vi "Keithley2450_and_24xx_plus_lockin_7_12_24.vi"() -> ()   [LabVIEW 2024]
uses:
  <vilib>/Analysis/1siggen.llb/Ramp Pattern by Delta.vi
  <vilib>/Utility/file.llb/Write Delimited Spreadsheet (string).vi
  <vilib>/Utility/file.llb/Write Delimited Spreadsheet (DBL).vi
  C:/Users/Public/OneDrive/Desktop/Keithley_2450_2470_1_4_0_LV2015_NewReadme2_2450-LV2015-1.4.0/Keithley 2450/Keithley 2450.lvlib
  <vilib>/Analysis/NI_AALBase.lvlib
  archive/Keithley 24XX/Keithley 24XX.lvlib
panel:
  out "XY Graph 2":cluster{dbl[], dbl[]}(graph)
  out "XY Graph":cluster{dbl[], dbl[]}(graph)
  in  "using 2400?":bool
  out "voltage 2410":dbl format="%0.2f"
  out "Current set voltage 2410":dbl
  in  "V stepsize 2410":dbl
  in  "start V 2410":dbl
  in  "End V 2410":dbl
  out "standard deviation current measured 2450":dbl=1.0551691053593696e-12 format="%0.5e"
  out "mean current measured 2450":dbl=3.19386155e-12 format="%0.5e"
  out "standard deviation current measured 2410":dbl format="%0.5e"
  out "mean current measured 2410":dbl format="%0.5e"
  in  "Compliance  Level 2410":dbl=1e-06
  in  "VISA resource name 2410":refnum<visa-resource-name>="GPIB0::24::INSTR"
  in  "Serial Configuration":T1={"Baud Rate"=9600, "Parity"=0, "Data Bits"=8, "Stop Bits"=10, "Flow Control"=0} {"Flow Control" items=["None", "XON/XOFF", "RTS/CTS", "XON/XOFF & RTS/CTS", "DTR/DSR", "XON/XOFF & DTR/DSR"]; "Stop Bits" items=["1.0"=10, "1.5"=15, "2.0"=20]; "Data Bits" items=["7"=7, "8"=8]; "Parity" items=["None", "Odd", "Even", "Mark", "Space"]; "Baud Rate" items=["300"=300, "600"=600, "1200"=1200, "2400"=2400, "4800"=4800, "9600"=9600, "19200"=19200]}
  in  "Wait for Current Meas":u32=100
  in  "Number of Current Meas":u32=20
  in  "Loop?":bool=TRUE
  out "Current set voltage 2450":dbl
  in  "V stepsize 2450":dbl=0.5
  in  "start V 2450":dbl
  in  "End V 2450":dbl=2.0
  in  "Wait for lock in meas (ms)":i32=2000
  in  "File Path":path=path "C:/Users/Public/OneDrive/Desktop/test.txt"
  out "错误输出":errorcluster={"status"=FALSE, "code"=1073676294, "source"="VISA Read in OE1022D_Query_Data.vi->Keithley2450_plus_lockin.vi"}
  out "Channel AWaveform Chart":dbl(graph)
  in  "Channel A Waveform Display":string(combo)="A-R"
  in  "Channel B Waveform Display":string(combo)="Channel_B_Rh1"
  out "Channel B Waveform Chart":dbl(graph)
  out "AUX-ADC4 (V)":sgl=0.009155273 format="%.3f"
  out "AUX-ADC3 (V)":sgl=0.010375977 format="%.3f"
  out "AUX-ADC1 (V)":sgl=0.0036621094 format="%.3f"
  out "AUX-ADC2 (V)":sgl=0.010986328 format="%.3f"
  out "R":sgl=0.008086495 caption="R (Vrms)" format="%.3p"
  out "X":sgl=0.008086206 caption="X (Vrms)" format="%.3p"
  out "Y":sgl=6.827377e-05 caption="Y (Vrms)" format="%.3p"
  out "θ (°)":sgl=0.4837504 caption="θ (deg)" format="%.2f"
  out "频率 (Hz)":sgl=6272.98 caption="Freq (Hz)" format="%#.3f"
  out "噪声":sgl=1.3872497e-05 caption="Noise(Vrms)" format="%.3p"
  out "Rh1":sgl=0.00035609925 caption="Rh1 (Vrms)" format="%.3p"
  out "θh1 (°)":sgl=-96.80644 caption="θh1 (deg)" format="%.2f"
  out "Xh1":sgl=-4.220333e-05 caption="Xh1 (Vrms)" format="%.3p"
  out "Yh1":sgl=-0.00035358954 caption="Yh1 (Vrms)" format="%.3p"
  out "X 2":sgl=7.4194313e-06 caption="X (Vrms)" format="%.3p"
  out "Y 2":sgl=-2.553077e-07 caption="Y (Vrms)" format="%.3p"
  out "R 2":sgl=7.423823e-06 caption="R (Vrms)" format="%.3p"
  out "θ (°) 2":sgl=-1.9708091 caption="θ (deg)" format="%.2f"
  out "频率 (Hz) 2":sgl=50064.324 caption="Freq (Hz)" format="%#.3f"
  out "噪声 2":sgl=1.4949475e-07 caption="Noise(Vrms)" format="%.3p"
  out "Xh1 2":sgl=-1.0919244e-06 caption="Xh1 (Vrms)" format="%.3p"
  out "Yh1 2":sgl=-0.00024940487 caption="Yh1 (Vrms)" format="%.3p"
  out "Rh1 2":sgl=0.00024940725 caption="Rh1 (Vrms)" format="%.3p"
  out "θh1 (°) 2":sgl=-90.25085 caption="θh1 (deg)" format="%.2f"
  in  "A Sensitivity":u16(ring)=22 items=["1 nV/fA", "2 nV/fA", "5 nV/fA", "10 nV/fA", "20 nV/fA", "50 nV/fA", "100 nV/fA", "200 nV/fA", "500 nV/fA", "1 uV/pA", "2 uV/pA", "5 uV/pA", "10 uV/pA", "20 uV/pA", "50 uV/pA", "100 uV/pA", "200 uV/pA", "500 uV/pA", "1 mV/nA", "2 mV/nA", "5 mV/nA", "10 mV/nA", "20 mV/nA", "50 mV/nA", "100 mV/nA", "200 mV/nA", "500 mV/nA", "1 V/uA"]
  in  "B Sensitivity":u16(ring)=18 items=["1 nV/fA", "2 nV/fA", "5 nV/fA", "10 nV/fA", "20 nV/fA", "50 nV/fA", "100 nV/fA", "200 nV/fA", "500 nV/fA", "1 uV/pA", "2 uV/pA", "5 uV/pA", "10 uV/pA", "20 uV/pA", "50 uV/pA", "100 uV/pA", "200 uV/pA", "500 uV/pA", "1 mV/nA", "2 mV/nA", "5 mV/nA", "10 mV/nA", "20 mV/nA", "50 mV/nA", "100 mV/nA", "200 mV/nA", "500 mV/nA", "1 V/uA"]
  out "序列号":string="SSI LIA-OE1022D,SN:D6712164,Ver6.3200831"
  in  "Num Lock in Points":i32=100
  in  "OE1022D":refnum<visa-resource-name>="COM6"
  in  "Current Compliance Limit (0.1) 2450":dbl=5e-08
  in  "VISA resource name 2450":refnum<visa-resource-name>="GPIB0::1::INSTR"
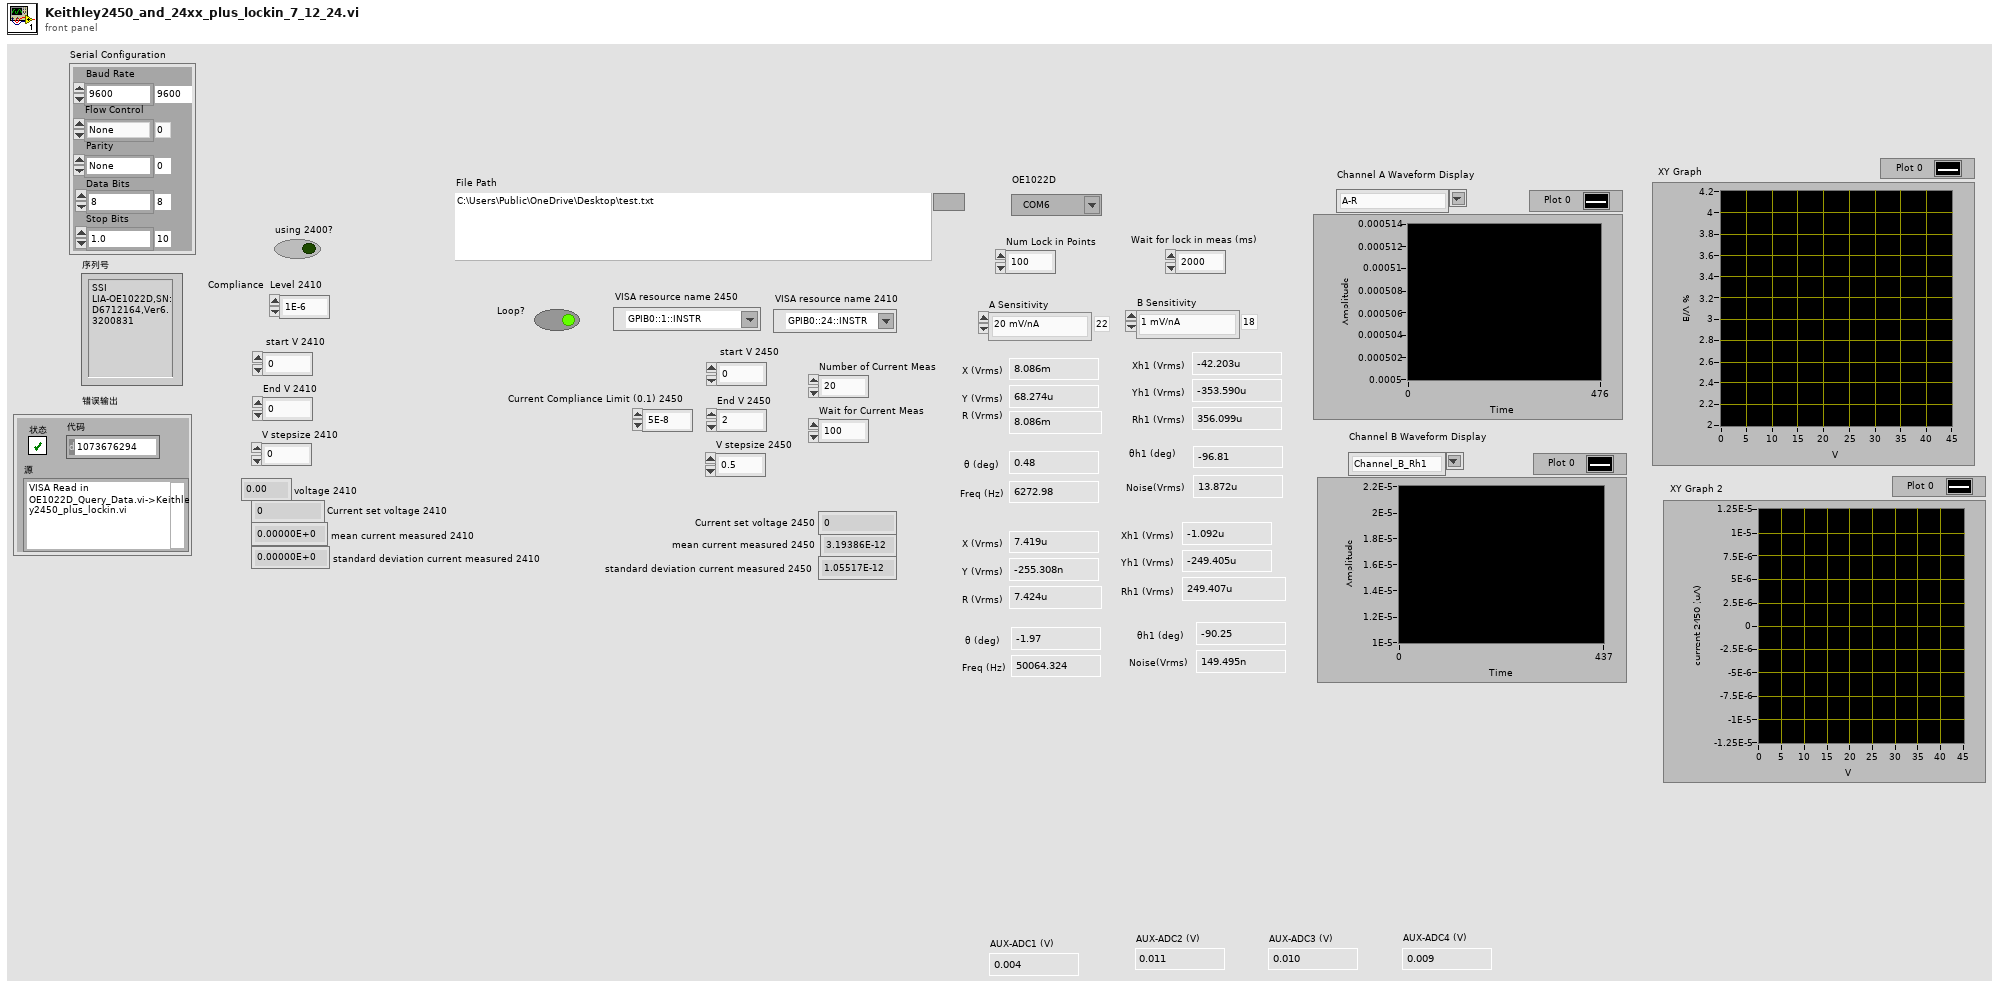
[diagram p1: front panel]
types:
  T1 = cluster{"Baud Rate":u32, "Parity":u16, "Data Bits":u16, "Stop Bits":u16, "Flow Control":u16}
  T2 = cluster{"AD1":dbl[], "AD2":dbl[], "AD3":dbl[], "AD4":dbl[]}
  T3 = cluster{"XB":dbl[], "YB":dbl[], "FrequencyB":dbl[], "NoiseB":dbl[], "Xh1B":dbl[], "Yh1B":dbl[], "Xh2B":dbl[], "Yh2B":dbl[], "Xh2B":dbl[]}
  T4 = cluster{"XA":dbl[], "YA":dbl[], "FrequencyA":dbl[], "NoiseA":dbl[], "Xh1A":dbl[], "Yh1A":dbl[], "Xh2A":dbl[], "Yh2A":dbl[]}
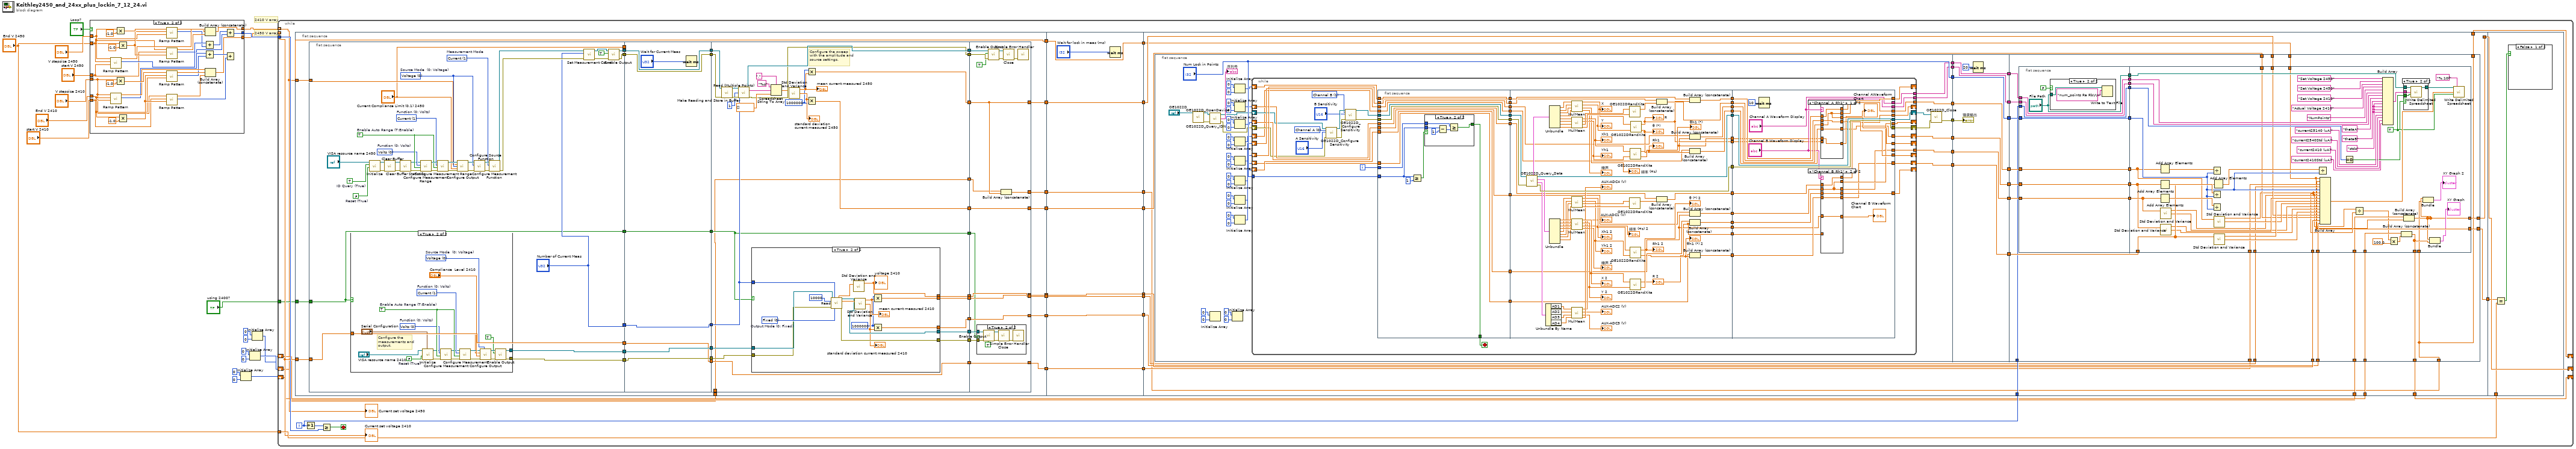
[diagram p0: block diagram]
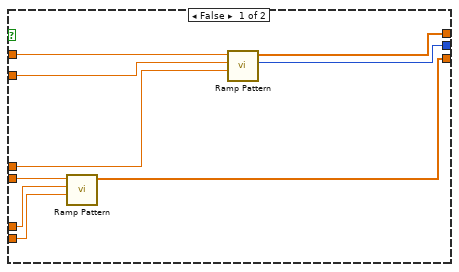
[diagram p2: hidden frame]
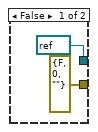
[diagram p3: hidden frame]
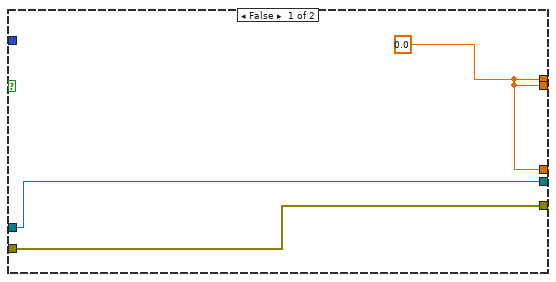
[diagram p4: hidden frame]
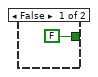
[diagram p6: hidden frame]
diagram:
  # "2410 V array"
  # "2450 V array"
  n1 = case shown="True" "Loop?" {
    tunnel: [w26 w53] -> w20
    tunnel: [w25 w48] -> w19
    tunnel: "V stepsize 2450" -> [w27 w47]
    tunnel: "start V 2450" -> [w28 w46]
    tunnel: "End V 2450" -> [w29 w45]
    tunnel: "End V 2410" -> [w24 w33]
    tunnel: "V stepsize 2410" -> [w22 w31]
    tunnel: "start V 2410" -> [w23 w32]
    tunnel: [w21 w30] -> w11
    frame False {
      n2 = call-poly <vilib>:"Ramp Pattern.vi"("start"=w23, "end"=w24, "delta"=w22) -> ("Ramp Pattern"=w21:dbl[])  [unwired: 6 in, 2 out]
      n3 = call-poly <vilib>:"Ramp Pattern.vi"("start"=w28, "end"=w29, "delta"=w27) -> ("samples"=w25:i32, "Ramp Pattern"=w26:dbl[])  [unwired: 6 in, 1 out]
    }
    frame True {
      n4 = call-poly <vilib>:"Ramp Pattern.vi"("start"=w46, "end"=w45, "delta"=w47) -> ("samples"=w52:i32, "Ramp Pattern"=w56:dbl[])  [unwired: 6 in, 1 out]
      n5 = call-poly <vilib>:"Ramp Pattern.vi"("start"=w32, "end"=w33, "delta"=w31) -> ("samples"=w37:i32, "Ramp Pattern"=w40:dbl[])  [unwired: 6 in, 1 out]
      n6 = Multiply(x=w47, y=-1.0) -> (x*y=w58:dbl)
      n7 = Multiply(x=w31, y=-1.0) -> (x*y=w42:dbl)
      n8 = Multiply(x=w45, y=-1.0) -> (x*y=w57:dbl)
      n9 = Multiply(x=w33, y=-1.0) -> (x*y=w41:dbl)
      n10 = call-poly <vilib>:"Ramp Pattern.vi"("start"=w45, "end"=w57, "delta"=w58) -> ("samples"=w51:i32, "Ramp Pattern"=w55:dbl[])  [unwired: 6 in, 1 out]
      n11 = call-poly <vilib>:"Ramp Pattern.vi"("start"=w57, "end"=w46, "delta"=w47) -> ("samples"=w50:i32, "Ramp Pattern"=w54:dbl[])  [unwired: 6 in, 1 out]
      n12 = call-poly <vilib>:"Ramp Pattern.vi"("start"=w33, "end"=w41, "delta"=w42) -> ("samples"=w36:i32, "Ramp Pattern"=w39:dbl[])  [unwired: 6 in, 1 out]
      n13 = call-poly <vilib>:"Ramp Pattern.vi"("start"=w41, "end"=w32, "delta"=w31) -> ("samples"=w35:i32, "Ramp Pattern"=w38:dbl[])  [unwired: 6 in, 1 out]
      n14 = Add(x=w52, y=w51) -> (x+y=w49:i32)
      n15 = Add(x=w37, y=w36) -> (x+y=w34:i32)
      n16 = Build Array (concatenate)(w56, w55, w54) -> (w53:dbl[])
      n17 = Build Array (concatenate)(w40, w39, w38) -> (w30:dbl[])
      n18 = Add(x=w49, y=w50) -> (x+y=w48:i32)
      n19 = Add(x=w34, y=w35) -> ()  [unwired: 1 out]
    }
  }
  n20 = Initialize Array(0, 0) -> (w7:i32[])
  n21 = Initialize Array(0, 0) -> (w4:i32[])
  n22 = Initialize Array(0, 0) -> (w1:i32[])
  n23 = while {
    tunnel: w20 -> [w61] mode=indexing
    tunnel: w19 -> [w91]
    tunnel: "End V 2450" -> [w84]
    tunnel: w11 -> [w71] mode=indexing
    tunnel: "using 2400?" -> [w70]
    shift-right: [w68] -> _
    shift-left: w7 -> [w69]
    shift-right: [w67] -> _
    shift-left: w4 -> [w66]
    shift-right: [w62] -> _
    shift-left: w1 -> [w65]
    i -> [w86]
    stop <- w90 stop-if-true
    n24 = flat-sequence {
      tunnel: w61 -> [w129]
      tunnel: [w129] -> w88
      tunnel: [w111] -> w82
      tunnel: [w110] -> w80
      tunnel: [w109] -> w78
      tunnel: [w108] -> w76
      tunnel: [w106] -> w74
      tunnel: [w102] -> w73
      tunnel: w71 -> [w101]
      tunnel: w70 -> [w98]
      tunnel: w65 -> [w93]
      tunnel: [w92] -> w63
      tunnel: w88 -> [w272]
      tunnel: [w272] -> w87
      tunnel: [w271] -> w83
      tunnel: w82 -> [w271]
      tunnel: [w270] -> w81
      tunnel: w80 -> [w270]
      tunnel: [w269] -> w79
      tunnel: w78 -> [w269]
      tunnel: [w268] -> w77
      tunnel: w76 -> [w268]
      tunnel: [w267] -> w75
      tunnel: w74 -> [w267]
      tunnel: w73 -> [w266]
      tunnel: [w266] -> w72
      tunnel: [w265] -> w64
      tunnel: w63 -> [w265]
      tunnel: w87 -> [w280]
      tunnel: w86 -> [w288]
      tunnel: [w287] -> w85
      tunnel: w83 -> [w282]
      tunnel: w81 -> [w281]
      tunnel: w79 -> [w286]
      tunnel: w77 -> [w285]
      tunnel: w75 -> [w284]
      tunnel: w72 -> [w283]
      tunnel: w69 -> [w279]
      tunnel: [w278] -> w68
      tunnel: [w277] -> w67
      tunnel: w66 -> [w276]
      tunnel: w64 -> [w275]
      tunnel: [w274] -> w62
      tunnel: w85 -> [w661]
      tunnel: w84 -> [w662]
      frame #0 {
        n25 = flat-sequence {
          tunnel: w129 -> [w149]
          tunnel: [w148] -> w128
          tunnel: ["Current Compliance Limit (0.1) 2450"] -> w126
          tunnel: [w146] -> w125
          tunnel: [w145] -> w123
          tunnel: [w144] -> w122
          tunnel: ["Number of Current Meas"] -> w116
          tunnel: [w138] -> w104
          tunnel: w101 -> [w138]
          tunnel: w98 -> [w130]
          tunnel: [w130] -> w96
          tunnel: w128 -> [w195]
          tunnel: [w195] -> w127
          tunnel: w126 -> [_]
          tunnel: w125 -> [w194]
          tunnel: [w194] -> w124
          tunnel: w123 -> [w192]
          tunnel: w122 -> [w191]
          tunnel: [w192] -> w121
          tunnel: [w191] -> w120
          tunnel: [w190] -> w117
          tunnel: w116 -> [w190]
          tunnel: [w189] -> w105
          tunnel: w104 -> [w189]
          tunnel: [w188] -> w97
          tunnel: w96 -> [w188]
          tunnel: w127 -> [w219]
          tunnel: w124 -> [w207]
          tunnel: w121 -> [w223]
          tunnel: w120 -> [w222]
          tunnel: [w221] -> w119
          tunnel: [w220] -> w118
          tunnel: w117 -> [w216]
          tunnel: [w210] -> w115
          tunnel: [w209] -> w114
          tunnel: [w200] -> w113
          tunnel: [w202] -> w112
          tunnel: [w205] -> w107
          tunnel: w105 -> [w206]
          tunnel: [w206] -> w103
          tunnel: [w204] -> w100
          tunnel: [w203] -> w99
          tunnel: w97 -> [w197]
          tunnel: [w197] -> w95
          tunnel: [w196] -> w94
          tunnel: w93 -> [w196]
          tunnel: w119 -> [w258]
          tunnel: w118 -> [w257]
          tunnel: w115 -> [w256]
          tunnel: w114 -> [w255]
          tunnel: w113 -> [w244]
          tunnel: w112 -> [w250]
          tunnel: [w244] -> w111
          tunnel: [w250] -> w110
          tunnel: [w249] -> w109
          tunnel: [w248] -> w108
          tunnel: [w247] -> w106
          tunnel: w107 -> [w247]
          tunnel: w103 -> [w246]
          tunnel: [w246] -> w102
          tunnel: w100 -> [w248]
          tunnel: w99 -> [w249]
          tunnel: w95 -> [w245]
          tunnel: w94 -> [w243]
          tunnel: [w242] -> w92
          frame #0 {
            w150 = u16 0 items=["Voltage", "Current"]  # Source Mode  (0: Voltage)
            w151 = u16 1 items=["Volts", "Current", "Auto Resistance", "Manual Resistance", "Digitize Voltage", "Digitize Current"]  # Measurement Mode
            w155 = TRUE  # Enable Auto Range (T:Enable)
            w153 = u16 1 items=["Volts", "Current", "Resistance"]  # Function (0: Volts)
            w154 = u16 0 items=["Volts", "Current", "Resistance"]  # Function (0: Volts)
            w137 = FALSE  # Reset (True)
            w156 = TRUE  # ID Query (True)
            n26 = case shown="True" w130 {
              tunnel: [refnum<visa-resource-name> refnum ("VISA resource name out") w174] -> w145
              tunnel: [errorcluster {"status"=FALSE, "code"=0, "source"=""} ("error out") w173] -> w144
              tunnel: w138 -> [_ w169]
              frame False {
              }
              frame True {
                w168 = FALSE  # Reset (True)
                w170 = u16 0 items=["Voltage", "Current"]  # Source Mode  (0: Voltage)
                w187 = TRUE  # Enable Auto Range (T:Enable)
                w183 = u16 1 items=["Volts", "Current", "Resistance"]  # Function (0: Volts)
                w182 = u16 0 items=["Volts", "Current", "Resistance"]  # Function (0: Volts)
                # "Configure the measurements and output."
                n27 = call "Initialize.vi"("Serial Configuration"="Serial Configuration", "Reset (True)"=w168, "VISA resource name"="VISA resource name 2410") -> ("error out"=w176:errorcluster, "VISA resource name out"=w175:refnum<visa-resource-name>)  [unwired: 7 in]
                n28 = call "Configure Measurement.vi"("error in (no error)"=w176, "Enable Auto Range (T:Enable)"=w187, "Function (0: Volts)"=w182, "VISA resource name"=w175) -> ("error out"=w177:errorcluster, "VISA resource name out"=w178:refnum<visa-resource-name>)  [unwired: 6 in]
                n29 = call "Configure Measurement.vi"("error in (no error)"=w177, "Enable Auto Range (T:Enable)"=w187, "Function (0: Volts)"=w183, "VISA resource name"=w178) -> ("error out"=w171:errorcluster, "VISA resource name out"=w172:refnum<visa-resource-name>)  [unwired: 6 in]
                n30 = call "Configure Output.vi"("Source Mode  (0: Voltage)"=w170, "error in (no error)"=w171, "Compliance  Level (0.1)"="Compliance  Level 2410", "Output Level (0)"=w169, "VISA resource name"=w172) -> ("error out"=w186:errorcluster, "VISA resource name out"=w185:refnum<visa-resource-name>)  [unwired: 5 in]
                n31 = call "Enable Output.vi"("error in (no error)"=w186, "Enable Output (T: Enable)"=TRUE, "VISA resource name"=w185) -> ("error out"=w173:errorcluster, "VISA resource name out"=w174:refnum<visa-resource-name>)  [unwired: 7 in]
              }
            }
            n32 = call "Initialize.vi"("Reset (True)"=w137, "ID Query (True)"=w156, "VISA resource name"="VISA resource name 2450") -> ("error out"=w135:errorcluster, "VISA resource name out"=w136:refnum<visa-resource-name>)  [unwired: 7 in]
            n33 = call "Clear Buffer.vi"("VISA resource name"=w136, "error in (no error)"=w135) -> ("VISA resource name out"=w134:refnum<visa-resource-name>, "error out"=w131:errorcluster)  [unwired: 12 in]
            n34 = call "Clear Buffer Statistics.vi"("VISA resource name"=w134, "error in (no error)"=w131) -> ("VISA resource name out"=w133:refnum<visa-resource-name>, "error out"=w132:errorcluster)  [unwired: 12 in]
            n35 = call "Configure Measurement Range.vi"("error in (no error)"=w132, "Enable Auto Range (T:Enable)"=w155, "Function (0: Volts)"=w154, "VISA resource name"=w133) -> ("error out"=w158:errorcluster, "VISA resource name out"=w157:refnum<visa-resource-name>)  [unwired: 6 in]
            n36 = call "Configure Measurement Range.vi"("error in (no error)"=w158, "Enable Auto Range (T:Enable)"=w155, "Function (0: Volts)"=w153, "VISA resource name"=w157) -> ("error out"=w163:errorcluster, "VISA resource name out"=w164:refnum<visa-resource-name>)  [unwired: 6 in]
            n37 = call "Configure Output.vi"("VISA resource name"=w164, "Source Level (0)"=w149, "Source Mode  (0: Voltage)"=w150, "Source Limit Level (0.1)"="Current Compliance Limit (0.1) 2450", "error in (no error)"=w163) -> ("VISA resource name out"=w159:refnum<visa-resource-name>, "error out"=w160:errorcluster)  [unwired: 9 in]
            n38 = call "Configure Source Function.vi"("error in (no error)"=w160, "Function (0: Volts)"=w150, "VISA resource name"=w159) -> ("error out"=w161:errorcluster, "VISA resource name out"=w162:refnum<visa-resource-name>)  [unwired: 7 in]
            n39 = call "Configure Measurement Function.vi"("error in (no error)"=w161, "Function (0: Volts)"=w151, "VISA resource name"=w162) -> ("error out"=w142:errorcluster, "VISA resource name out"=w143:refnum<visa-resource-name>)  [unwired: 7 in]
            n40 = call "Set Measurement Count.vi"("error in (no error)"=w142, "Measurement Count"="Number of Current Meas", "VISA resource name"=w143) -> ("error out"=w141:errorcluster, "VISA resource name out"=w140:refnum<visa-resource-name>)  [unwired: 7 in]
            n41 = call "Enable Output.vi"("error in (no error)"=w141, "Enable Output (T: Enable)"=TRUE, "VISA resource name"=w140) -> ("error out"=w146:errorcluster, "VISA resource name out"=w148:refnum<visa-resource-name>)  [unwired: 7 in]
          }
          frame #1 {
            n42 = Wait (ms)(milliseconds to wait="Wait for Current Meas") -> ()  [unwired: 1 out]
          }
          frame #2 {
            w198 = 1000000 ("Timeout (10000 ms)")
            # "Configure the sweep with the amplitude and source settings."
            n43 = call "Make Reading and Store in Buffer.vi"("VISA resource name"=w219, "error in (no error)"=w207) -> ("VISA resource name out"=w217:refnum<visa-resource-name>, "error out"=w218:errorcluster)  [unwired: 12 in]
            n44 = call "Read (Multiple Points).vi"("VISA resource name"=w217, "Start Index (1)"=u32 1, "End Index (1)"=w216, "error in (no error)"=w218) -> ("VISA resource name out"=w210:refnum<visa-resource-name>, "Data out"=w211:string, "error out"=w209:errorcluster)  [unwired: 9 in]
            n45 = case shown="True" w197 {
              tunnel: w223 -> [w226 w238]
              tunnel: w222 -> [w225 w237]
              tunnel: [w225 w236] -> w221
              tunnel: [w226 w235] -> w220
              tunnel: w216 -> [_ w234]
              tunnel: [w224 w232] -> w205
              tunnel: [w224 w231] -> w204
              tunnel: [w224 w228] -> w203
              frame False {
                w224 = 0.0 ("mean")
              }
              frame True {
                w227 = 1000000 ("Timeout (10000 ms)")
                w240 = u16 0 items=["Fixed", "Sweep", "List"]  # Output Mode (0: Fixed)
                n46 = call-poly "Read.vi"("VISA resource name"=w238, "Sample Count (1)"=w234, "Timeout (10000 ms)"=10000, "error in (no error)"=w237, "Output Mode (0: Fixed)"=w240) -> ("Voltage"=w233:sgl[], "VISA resource name out"=w235:refnum<visa-resource-name>, "Current"=w239:sgl[], "error out"=w236:errorcluster)  [unwired: 4 in, 3 out]
                n47 = call <vilib>:"Std Deviation and Variance.vi"("X"=w233) -> ("mean"=w232:dbl)  [unwired: 1 in, 2 out]
                "voltage 2410" <- w232
                n48 = call <vilib>:"Std Deviation and Variance.vi"("X"=w239) -> ("mean"=w229:dbl, "standard deviation"=w230:dbl)  [unwired: 1 in, 1 out]
                "mean current measured 2410" <- w229
                "standard deviation current measured 2410" <- w230
                n49 = Multiply(x=w227, y=w229) -> (x*y=w228:dbl)
                n50 = Multiply(x=w227, y=w230) -> (x*y=w231:dbl)
              }
            }
            n51 = Spreadsheet String To Array(delimiter (Tab)=",", format string="%s", spreadsheet string=w211, array type (2D Dbl)=dbl[] []) -> (array=w208:dbl[])
            n52 = call <vilib>:"Std Deviation and Variance.vi"("X"=w208) -> ("mean"=w199:dbl, "standard deviation"=w201:dbl)  [unwired: 1 in, 1 out]
            "mean current measured 2450" <- w199
            "standard deviation current measured 2450" <- w201
            n53 = Multiply(x=w198, y=w199) -> (x*y=w200:dbl)
            n54 = Multiply(x=w201, y=w198) -> (x*y=w202:dbl)
          }
          frame #3 {
            n55 = case shown="True" w245 {
              tunnel: w258 -> [_ w264]
              tunnel: w257 -> [_ w263]
              frame False {
              }
              frame True {
                n56 = call "Enable Output.vi"("error in (no error)"=w264, "Enable Output (T: Enable)"=TRUE, "VISA resource name"=w263) -> ("error out"=w261:errorcluster, "VISA resource name out"=w262:refnum<visa-resource-name>)  [unwired: 7 in]
                n57 = call "Close.vi"("error in (no error)"=w261, "VISA resource name"=w262) -> ("error out"=w260:errorcluster)  [unwired: 9 in]
                n58 = call <vilib>:"Simple Error Handler.vi"("error in (no error)"=w260) -> ()  [unwired: 4 in, 5 out]
              }
            }
            n59 = call "Enable Output.vi"("error in (no error)"=w255, "Enable Output (T: Enable)"=TRUE, "VISA resource name"=w256) -> ("error out"=w252:errorcluster, "VISA resource name out"=w253:refnum<visa-resource-name>)  [unwired: 7 in]
            n60 = Build Array (concatenate)(w243, w244) -> (w242:dbl[])
            n61 = call "Close.vi"("error in (no error)"=w252, "VISA resource name"=w253) -> ("error out"=w251:errorcluster)  [unwired: 9 in]
            n62 = call <vilib>:"Simple Error Handler.vi"("error in (no error)"=w251) -> ()  [unwired: 4 in, 5 out]
          }
        }
      }
      frame #1 {
        n63 = Wait (ms)(milliseconds to wait="Wait for lock in meas (ms)") -> ()  [unwired: 1 out]
      }
      frame #2 {
        n64 = flat-sequence {
          tunnel: [w324] -> w303
          tunnel: [w323] -> w302
          tunnel: ["Num Lock in Points"] -> w301
          tunnel: [w318] -> w300
          tunnel: [w322] -> w299
          tunnel: [w321] -> w298
          tunnel: [w308] -> w297
          tunnel: [w309] -> w296
          tunnel: w303 -> [w558]
          tunnel: [w558] -> w295
          tunnel: w302 -> [w557]
          tunnel: [w557] -> w294
          tunnel: w301 -> [w556]
          tunnel: [w556] -> w293
          tunnel: w300 -> [w554]
          tunnel: [w553] -> w292
          tunnel: w299 -> [w553]
          tunnel: w298 -> [w552]
          tunnel: [w552] -> w291
          tunnel: [w551] -> w290
          tunnel: w297 -> [w551]
          tunnel: w296 -> [w550]
          tunnel: [w550] -> w289
          tunnel: w295 -> [w583]
          tunnel: w294 -> [w582]
          tunnel: w293 -> [w581]
          tunnel: w292 -> [w579]
          tunnel: w291 -> [w578]
          tunnel: w290 -> [w576]
          tunnel: w289 -> [w574]
          tunnel: w288 -> [w572]
          tunnel: [w571] -> w287
          tunnel: w286 -> [w570]
          tunnel: w285 -> [w569]
          tunnel: w284 -> [w567]
          tunnel: w283 -> [w568]
          tunnel: w282 -> [w566]
          tunnel: w281 -> [w565]
          tunnel: w280 -> [w564]
          tunnel: w279 -> [w563]
          tunnel: [w562] -> w278
          tunnel: [w561] -> w277
          tunnel: w276 -> [w560]
          tunnel: w275 -> [w559]
          tunnel: [w559] -> w274
          frame #0 {
            n65 = call "OE1022D_OpenDevice.vi"("VISA resource name"="OE1022D") -> ("VISA资源名称输出"=w346:refnum<visa-resource-name>, "错误输出"=w345:errorcluster)  [unwired: 17 in]
            n66 = call "OE1022D_Query_IDN.vi"("错误输入（无错误）"=w345, "VISA resource name"=w346) -> ("错误输出"=w316:errorcluster, "序列号"=→"序列号":string, "VISA resource name out"=w317:refnum<visa-resource-name>)  [unwired: 1 in]
            n67 = Initialize Array(0, 0) -> ()  [unwired: 1 out]
            n68 = Initialize Array(0, 0) -> ()  [unwired: 1 out]
            n69 = Initialize Array(0, 0) -> (w342:i32[])
            n70 = Initialize Array(0, 0) -> (w326:i32[])
            n71 = Initialize Array(0, 0) -> (w325:i32[])
            n72 = Initialize Array(0, 0) -> (w311:i32[])
            n73 = Initialize Array(0, 0) -> (w331:i32[])
            n74 = Initialize Array(0, 0) -> (w332:i32[])
            n75 = Initialize Array(0, 0) -> (w310:i32[])
            n76 = Initialize Array(0, 0) -> (w337:i32[])
            n77 = while {
              shift-right: [w403] -> _
              shift-left: w342 -> [w402]
              shift-right: [w400] -> _
              shift-left: w337 -> [w399]
              tunnel: "Num Lock in Points" -> [w392]
              shift-right: [w380] -> _
              shift-left: w331 -> [w382]
              shift-right: [w376] -> _
              shift-left: w332 -> [w379]
              shift-right: [w369] -> _
              shift-left: w325 -> [w375]
              shift-right: [w368] -> _
              shift-left: w326 -> [w374]
              tunnel: [w367] -> w324
              tunnel: [w366] -> w323
              tunnel: [w365] -> w322
              tunnel: [w364] -> w321
              shift-right: [w363] -> w320
              shift-left: w316 -> [w360]
              shift-right: [w362] -> w319
              shift-left: w317 -> [w361]
              shift-right: [w352] -> w308
              shift-left: w311 -> [w356]
              shift-right: [w353] -> w309
              shift-left: w310 -> [w354]
              i -> [w394]
              stop <- w393 stop-if-true
              w385 = u8 1 items=["Channel A", "Channel B"] ("OE1022D A/B")
              w391 = u8 0 items=["Channel A", "Channel B"] ("OE1022D A/B")
              n78 = call "OE1022D_Configure Sensitivity.vi"("VISA resource name"=w361, "OE1022D A/B"=w391, "Sensitivity"="A Sensitivity", "error in (no error)"=w360) -> ("VISA resource name out"=w386:refnum<visa-resource-name>, "error out"=w387:errorcluster)  [unwired: 14 in]
              n79 = call "OE1022D_Configure Sensitivity.vi"("VISA resource name"=w386, "OE1022D A/B"=w385, "Sensitivity"="B Sensitivity", "error in (no error)"=w387) -> ("VISA resource name out"=w389:refnum<visa-resource-name>, "error out"=w388:errorcluster)  [unwired: 14 in]
              n80 = flat-sequence {
                tunnel: w399 -> [w418]
                tunnel: w402 -> [w419]
                tunnel: w389 -> [w420]
                tunnel: w388 -> [w421]
                tunnel: [w421] -> w398
                tunnel: [w420] -> w397
                tunnel: [w419] -> w396
                tunnel: [w418] -> w395
                tunnel: w394 -> [w417]
                tunnel: [w416] -> w393
                tunnel: w392 -> [w414]
                tunnel: [w412] -> w383
                tunnel: w382 -> [w412]
                tunnel: w379 -> [w411]
                tunnel: [w411] -> w378
                tunnel: w375 -> [w410]
                tunnel: w374 -> [w409]
                tunnel: [w410] -> w373
                tunnel: [w409] -> w372
                tunnel: [w408] -> w357
                tunnel: w356 -> [w408]
                tunnel: [w407] -> w355
                tunnel: w354 -> [w407]
                tunnel: [w498] -> w406
                tunnel: [w497] -> w405
                tunnel: [w451] -> w404
                tunnel: [w448] -> w401
                tunnel: w398 -> [w500]
                tunnel: w397 -> [w499]
                tunnel: w396 -> [w452]
                tunnel: w395 -> [w450]
                tunnel: w383 -> [w447]
                tunnel: [w446] -> w381
                tunnel: w378 -> [w444]
                tunnel: [w443] -> w377
                tunnel: w373 -> [w440]
                tunnel: w372 -> [w441]
                tunnel: [w439] -> w371
                tunnel: [w438] -> w370
                tunnel: [w434] -> w359
                tunnel: [w436] -> w358
                tunnel: w357 -> [w433]
                tunnel: w355 -> [w432]
                tunnel: [w431] -> w351
                tunnel: [w430] -> w350
                tunnel: [w429] -> w349
                tunnel: [w428] -> w348
                tunnel: w406 -> [w527]
                tunnel: w405 -> [w528]
                tunnel: w404 -> [w526]
                tunnel: [w524] -> w403
                tunnel: w401 -> [w520]
                tunnel: [w519] -> w400
                tunnel: [w528] -> w362
                tunnel: [w527] -> w363
                tunnel: w381 -> [w525]
                tunnel: [w523] -> w380
                tunnel: w377 -> [w522]
                tunnel: [w521] -> w376
                tunnel: w371 -> [w515]
                tunnel: w370 -> [w518]
                tunnel: [w517] -> w369
                tunnel: [w516] -> w368
                tunnel: [w514] -> w367
                tunnel: [w513] -> w366
                tunnel: ["Channel A Waveform Display"] -> w365
                tunnel: ["Channel B Waveform Display"] -> w364
                tunnel: w359 -> [w509]
                tunnel: [w508] -> w352
                tunnel: [w507] -> w353
                tunnel: w358 -> [w510]
                tunnel: w351 -> [w506]
                tunnel: w350 -> [w504]
                tunnel: w349 -> [w503]
                tunnel: w348 -> [w501]
                frame #0 {
                  n81 = Greater Or Equal?(x=w414, y=1) -> (x >= y?=w413:bool)
                  n82 = case shown="True" w413 {
                    tunnel: w417 -> [_ w427]
                    tunnel: [FALSE w426] -> w416
                    tunnel: w414 -> [_ w423]
                    frame False {
                    }
                    frame True {
                      n83 = Subtract(x=w423, y=1) -> (x-y=w424:i32)
                      n84 = Greater Or Equal?(x=w427, y=w424) -> (x >= y?=w426:bool)
                    }
                  }
                }
                frame #1 {
                  n85 = call "OE1022D_Query_Data.vi"("错误输入（无错误）"=w500, "VISA resource name"=w499) -> ("error out"=w498:errorcluster, "输出簇ADC"=w454:T2, "输出簇B"=w453:T3, "VISA resource name out"=w497:refnum<visa-resource-name>, "输出簇A"=w449:T4)  [unwired: 3 in]
                  n86 = Unbundle By Name(w454) -> ("AD1"=w493:dbl[], "AD2"=w494:dbl[], "AD3"=w495:dbl[], "AD4"=w496:dbl[])
                  n87 = Unbundle(w449) -> ("XA"=w459:dbl[], "YA"=w460:dbl[], "FrequencyA"=w461:dbl[], "NoiseA"=w462:dbl[], "Xh1A"=w467:dbl[], "Yh1A"=w468:dbl[], "Xh2A"=w469:dbl[], "Yh2A"=w470:dbl[])
                  n88 = Unbundle(w453) -> ("XB"=w483:dbl[], "YB"=w482:dbl[], "FrequencyB"=w481:dbl[], "NoiseB"=w480:dbl[], "Xh1B"=w479:dbl[], "Yh1B"=w478:dbl[], "Xh2B"=w477:dbl[], "Yh2B"=w476:dbl[])  [unwired: 1 out]
                  n89 = call "MulMean.vi"("IN 4"=w462, "IN 3"=w461, "IN 2"=w460, "IN 1"=w459) -> ("mean 4"=→"噪声":dbl, "mean 3"=→"频率 (Hz)":dbl, "mean 2"=w465:dbl, "mean 1"=w464:dbl)  [unwired: 4 in]
                  "X" <- w464
                  "Y" <- w465
                  n90 = call "MulMean.vi"("IN 4"=w470, "IN 3"=w469, "IN 2"=w468, "IN 1"=w467) -> ("mean 4"=w475:dbl, "mean 3"=w474:dbl, "mean 2"=w472:dbl, "mean 1"=w471:dbl)  [unwired: 4 in]
                  "Xh1" <- w471
                  "Yh1" <- w472
                  n91 = call "MulMean.vi"("IN 4"=w476, "IN 3"=w477, "IN 2"=w478, "IN 1"=w479) -> ("mean 4"=w492:dbl, "mean 3"=w491:dbl, "mean 2"=w490:dbl, "mean 1"=w489:dbl)  [unwired: 4 in]
                  "Xh1 2" <- w489
                  "Yh1 2" <- w490
                  n92 = call "MulMean.vi"("IN 4"=w480, "IN 3"=w481, "IN 2"=w482, "IN 1"=w483) -> ("mean 4"=→"噪声 2":dbl, "mean 3"=→"频率 (Hz) 2":dbl, "mean 2"=w488:dbl, "mean 1"=w487:dbl)  [unwired: 4 in]
                  "X 2" <- w487
                  "Y 2" <- w488
                  n93 = call "MulMean.vi"("IN 4"=w496, "IN 3"=w495, "IN 2"=w494, "IN 1"=w493) -> ("mean 4"=→"AUX-ADC4 (V)":dbl, "mean 3"=→"AUX-ADC3 (V)":dbl, "mean 2"=→"AUX-ADC2 (V)":dbl, "mean 1"=→"AUX-ADC1 (V)":dbl)  [unwired: 4 in]
                  n94 = call "OE1022DRandXita.vi"("Y"=w475, "X"=w474) -> ("R"=w445:dbl)  [unwired: 1 out]
                  n95 = call "OE1022DRandXita.vi"("Y"=w492, "X"=w491) -> ("R"=w442:dbl)  [unwired: 1 out]
                  n96 = call "OE1022DRandXita.vi"("Y"=w472, "X"=w471) -> ("θ (°)"=→"θh1 (°)":dbl, "R"=w428:dbl)
                  "Rh1" <- w428
                  n97 = call "OE1022DRandXita.vi"("Y"=w490, "X"=w489) -> ("θ (°)"=w437:dbl, "R"=w431:dbl)
                  "Rh1 2" <- w431
                  "θh1 (°) 2" <- w437
                  n98 = call "OE1022DRandXita.vi"("Y"=w488, "X"=w487) -> ("θ (°)"=→"θ (°) 2":dbl, "R"=w430:dbl)
                  "R 2" <- w430
                  n99 = call "OE1022DRandXita.vi"("Y"=w465, "X"=w464) -> ("θ (°)"=w435:dbl, "R"=w429:dbl)
                  "R" <- w429
                  "θ (°)" <- w435
                  n100 = Build Array (concatenate)(w444, w445) -> (w443:dbl[])
                  n101 = Build Array (concatenate)(w441, w442) -> (w438:dbl[])
                  n102 = Build Array (concatenate)(w452, w429) -> (w451:dbl[])
                  n103 = Build Array (concatenate)(w447, w428) -> (w446:dbl[])
                  n104 = Build Array (concatenate)(w433, w435) -> (w434:dbl[])
                  n105 = Build Array (concatenate)(w440, w431) -> (w439:dbl[])
                  n106 = Build Array (concatenate)(w450, w430) -> (w448:dbl[])
                  n107 = Build Array (concatenate)(w432, w437) -> (w436:dbl[])
                }
                frame #2 {
                  n108 = Wait (ms)(milliseconds to wait=10) -> ()  [unwired: 1 out]
                  n109 = case shown="\"Channel_A_Rh1\"" "Channel A Waveform Display" {
                    tunnel: w526 -> [w544 w547]
                    tunnel: [w544 w547] -> w524
                    tunnel: w525 -> [w542 w549]
                    tunnel: [w542 w549] -> w523
                    tunnel: w522 -> [w543 w548]
                    tunnel: [w543 w548] -> w521
                    tunnel: [w542 w547] -> w514
                    tunnel: w509 -> [w541 w546]
                    tunnel: [w541 w546] -> w508
                    tunnel: w503 -> [_ w545]
                    tunnel: [w540 w545] -> w502
                    tunnel: w501 -> [w540 _]
                    frame "Channel_A_Rh1" {
                    }
                    frame "Channel_A_R", Default {
                    }
                  }
                  "Channel AWaveform Chart" <- w502
                  n110 = case shown="\"Channel_B_Rh1\"" "Channel B Waveform Display" {
                    tunnel: [w534 w537] -> w513
                    tunnel: w520 -> [w534 w539]
                    tunnel: [w534 w539] -> w519
                    tunnel: w518 -> [w533 w538]
                    tunnel: [w533 w538] -> w516
                    tunnel: [w532 w537] -> w517
                    tunnel: w515 -> [w532 w537]
                    tunnel: w510 -> [w531 w536]
                    tunnel: [w531 w536] -> w507
                    tunnel: w506 -> [_ w535]
                    tunnel: [w530 w535] -> w505
                    tunnel: w504 -> [w530 _]
                    frame "Channel_B_R", Default {
                    }
                    frame "Channel_B_Rh1" {
                    }
                  }
                  "Channel B Waveform Chart" <- w505
                }
              }
            }
            n111 = call "OE1022D_Close.vi"("错误输入（无错误）"=w320, "VISA resource name"=w319) -> ("错误输出"=w318:errorcluster)  [unwired: 1 in]
          }
          frame #1 {
            n112 = Wait (ms)(milliseconds to wait=20) -> ()  [unwired: 1 out]
            "错误输出" <- w554
          }
          frame #2 {
            n113 = flat-sequence {
              tunnel: w581 -> [w594]
              tunnel: w582 -> [w595]
              tunnel: w583 -> [w596]
              tunnel: [w596] -> w587
              tunnel: [w595] -> w586
              tunnel: [w594] -> w585
              tunnel: ["File Path"] -> w584
              tunnel: [w591] -> w580
              tunnel: w579 -> [w591]
              tunnel: w578 -> [w590]
              tunnel: [w590] -> w577
              tunnel: w576 -> [w589]
              tunnel: [w589] -> w575
              tunnel: [w588] -> w573
              tunnel: w572 -> [w588]
              tunnel: w587 -> [w636]
              tunnel: w586 -> [w639]
              tunnel: w585 -> [w642]
              tunnel: w584 -> [w649]
              tunnel: w580 -> [w647]
              tunnel: w577 -> [w646]
              tunnel: w575 -> [w637]
              tunnel: w574 -> [w638]
              tunnel: w573 -> [w626]
              tunnel: [w608] -> w571
              tunnel: w570 -> [w624]
              tunnel: w569 -> [w623]
              tunnel: w568 -> [w620]
              tunnel: w567 -> [w619]
              tunnel: w566 -> [w613]
              tunnel: w565 -> [w612]
              tunnel: w564 -> [w608]
              tunnel: w563 -> [w609]
              tunnel: [w606] -> w562
              tunnel: [w601] -> w561
              tunnel: w560 -> [w607]
              tunnel: w559 -> [w600]
              frame #0 {
                n114 = case shown="True" FALSE {
                  tunnel: "File Path" -> [_ w598]
                  frame False {
                  }
                  frame True {
                    n115 = Write to Text File(file (use dialog)=w598, text="num_points Ra Rb\r\n") -> ()  [unwired: 2 in, 3 out]
                  }
                }
              }
              frame #1 {
                w629 = "stds"
                w648 = TRUE
                n116 = Add Array Elements(numeric array=w636) -> (sum=w653:dbl)
                n117 = Add Array Elements(numeric array=w637) -> (sum=w644:dbl)
                n118 = Add Array Elements(numeric array=w639) -> (sum=w651:dbl)
                n119 = call <vilib>:"Std Deviation and Variance.vi"("X"=w639) -> ("mean"=w611:dbl, "standard deviation"=w630:dbl)  [unwired: 1 in, 1 out]
                n120 = call <vilib>:"Std Deviation and Variance.vi"("X"=w637) -> ("mean"=w635:dbl, "standard deviation"=w632:dbl)  [unwired: 1 in, 1 out]
                n121 = Divide(x=w653, y=w642) -> ()  [unwired: 1 out]
                n122 = Divide(x=w644, y=w642) -> ()  [unwired: 1 out]
                n123 = Divide(x=w651, y=w642) -> ()  [unwired: 1 out]
                n124 = Add Array Elements(numeric array=w638) -> (sum=w643:dbl)
                n125 = call <vilib>:"Std Deviation and Variance.vi"("X"=w636) -> ("mean"=w610:dbl, "standard deviation"=w631:dbl)  [unwired: 1 in, 1 out]
                n126 = call <vilib>:"Std Deviation and Variance.vi"("X"=w638) -> ("mean"=w634:dbl, "standard deviation"=w633:dbl)  [unwired: 1 in, 1 out]
                n127 = Divide(x=w643, y=w642) -> ()  [unwired: 1 out]
                n128 = Build Array(w608, w608, w620, w619, w642, w610, w611, w635, w634, w631, w630, w632, w633, w613, w612, w624, w623) -> (w652:dbl[])
                n129 = Equal To 0?(x=w626) -> (x = 0?=w625:bool)
                n130 = Divide(x=w611, y=w610) -> (x/y=w603:dbl)
                n131 = Build Array("Set Voltage 2450", "Set Voltage 2450", "Set Voltage 2410", "Actual Voltage 2410", "NumPoints", w647, w646, "thetaA", "thetaB", w629, w629, w629, w629, "current25140 (uA)", "current2540Std (uA)", "current2410 (uA)", "current2410Std (uA)") -> (w645:string[])
                n132 = Multiply(x=w603, y=100.0) -> (x*y=w604:dbl)
                n133 = Build Array (concatenate)(w609, w604) -> (w606:dbl[])
                n134 = case shown="True" w625 {
                  tunnel: [w655 w659] -> w650
                  tunnel: w649 -> [w655 w658]
                  tunnel: w648 -> [_ w657]
                  tunnel: w645 -> [_ w656]
                  frame False {
                  }
                  frame True {
                    n135 = call-poly <vilib>:"Write Delimited Spreadsheet.vi"("file path (dialog if empty)"=w658, "1D data"=w656, "append to file? (new file:F)"=w657) -> ("new file path (Not A Path if cancelled)"=w659:path)  [unwired: 11 in, 1 out]
                  }
                }
                n136 = Build Array (concatenate)(w607, w608) -> (w601:dbl[])
                n137 = Bundle(w601, w600) -> (→"XY Graph 2":cluster{dbl[], dbl[]})  [unwired: 1 in]
                n138 = Bundle(w601, w606) -> (→"XY Graph":cluster{dbl[], dbl[]})  [unwired: 1 in]
                n139 = call-poly <vilib>:"Write Delimited Spreadsheet.vi"("file path (dialog if empty)"=w650, "format (%.3f)"="%.10f", "1D data"=w652, "append to file? (new file:F)"=w648) -> ()  [unwired: 10 in, 2 out]
              }
            }
          }
        }
      }
      frame #3 {
        n140 = Equal?(x=w661, y=w662) -> (x = y?=w660:bool)
        n141 = case shown="False" w660 {
          frame False {
          }
          frame True {
          }
        }
      }
    }
    n142 = Increment(x=w86) -> (x+1=w89:i32)
    n143 = Greater Or Equal?(x=w89, y=w91) -> (x >= y?=w90:bool)
    "Current set voltage 2450" <- w61
    "Current set voltage 2410" <- w71
  }
